vi "Operator_id_check.vi"(10 "Numeric 2":i32, 11 "in":bool) -> (2 "Numeric":i32, 3 "out":bool)   [LabVIEW 2021]
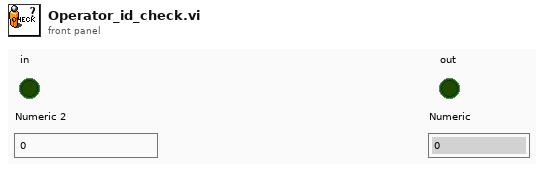
[diagram p1: front panel]
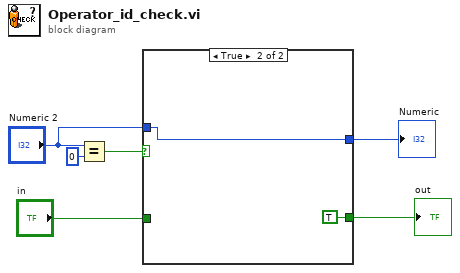
[diagram p0: block diagram]
diagram:
  n1 = Equal?(x="Numeric 2", y=0) -> (x = y?=w6:bool)
  n2 = case shown="True" w6 {
    tunnel: [w8 TRUE] -> w5
    tunnel: [w7 w9] -> w4
    tunnel: "Numeric 2" -> [w7 w9]
    tunnel: "in" -> [w8 _]
    frame False {
    }
    frame True {
    }
  }
  "Numeric" <- w4
  "out" <- w5
